vi "Calculate Cc.vi"(8 "error in":errorcluster, 11 "Particle Properties in":refnum<class "Particle Properties.lvclass">) -> (0 "error out":errorcluster, 2 "Cc":dbl, 3 "Particle Properties out":refnum<class "Particle Properties.lvclass">)   [LabVIEW 2015, in "Particle Properties.lvclass"]
doc: "Calculate the Cunningham correction factor following Hinds [1999], Aerosol Technology: Properties, Behavior and Measurement of Airbourne Particles."
uses:
  Particle Properties.lvclass
  Particle Properties.lvclass/Particle Properties.ctl
  Accessors/Read D.vi
  Accessors/Read Gas Ref.vi
  Atmospheric/Gas Properties/Gas Properties.lvclass
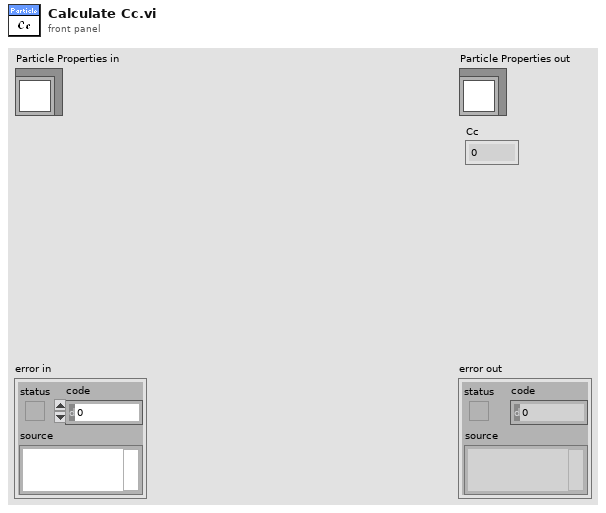
[diagram p1: front panel]
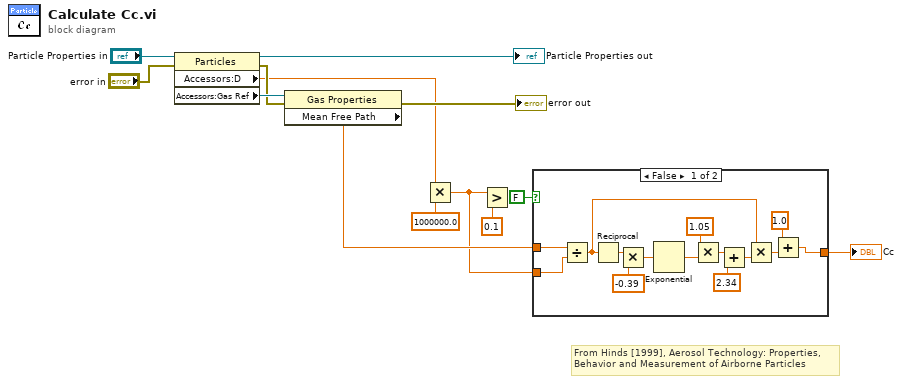
[diagram p0: block diagram]
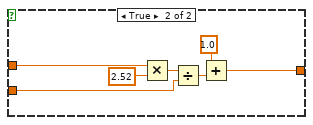
[diagram p2: hidden frame]
diagram:
  # "From Hinds [1999], Aerosol Technology: Properties, Behavior and Measurement of Airborne Particles"
  n1 = property class="Particles"(reference="Particle Properties in", error in="error in") -> (reference out=→"Particle Properties out":refnum<class "Particle Properties.lvclass">, error out=w6:errorcluster, "Accessors:D"=w3:dbl, "Accessors:Gas Ref"=w10:refnum<data-value>)
  n2 = property class="Gas Properties"(reference=w10, error in=w6) -> (error out=→"error out":errorcluster, "Mean Free Path"=w11:dbl)  [unwired: 1 out]
  n3 = Multiply(x=w3, y=1000000.0) -> (x*y=w2:dbl)
  n4 = Greater?(x=w2, y=0.1) -> ()  [unwired: 1 out]
  n5 = case shown="False" FALSE {
    tunnel: w11 -> [w26 w33]
    tunnel: w2 -> [w25 w30]
    tunnel: [w16 w28] -> w12
    frame False {
      n6 = Divide(x=w26, y=w25) -> (x/y=w14:dbl)
      n7 = Reciprocal(x=w14) -> (1/x=w21:dbl)
      n8 = Multiply(x=w21, y=-0.39) -> (x*y=w20:dbl)
      n9 = Exponential(1:w20) -> (0:w19:dbl)
      n10 = Multiply(x=1.05, y=w19) -> (x*y=w18:dbl)
      n11 = Add(x=w18, y=2.34) -> (x+y=w15:dbl)
      n12 = Multiply(x=w14, y=w15) -> (x*y=w17:dbl)
      n13 = Add(x=1.0, y=w17) -> (x+y=w16:dbl)
    }
    frame True {
      n14 = Multiply(x=w33, y=2.52) -> (x*y=w31:dbl)
      n15 = Divide(x=w31, y=w30) -> (x/y=w29:dbl)
      n16 = Add(x=1.0, y=w29) -> (x+y=w28:dbl)
    }
  }
  "Cc" <- w12
